vi "Coordinate RND.vi"(8 "Coordinate Min":dbl=10.0, 9 "Coordinate Max":dbl=15.0, 11 "City's":u16=3) -> (1 "City's":cluster{"X":dbl, "Y":dbl}[](graph), 3 "Coordinate[]":T1[](array[typedef]))   [LabVIEW 2015, in "TSP Library.lvlib"]
uses:
  TSP Library.lvlib
  TypeDef/Coordinate.ctl
  <vilib>/Analysis/NI_AALBase.lvlib
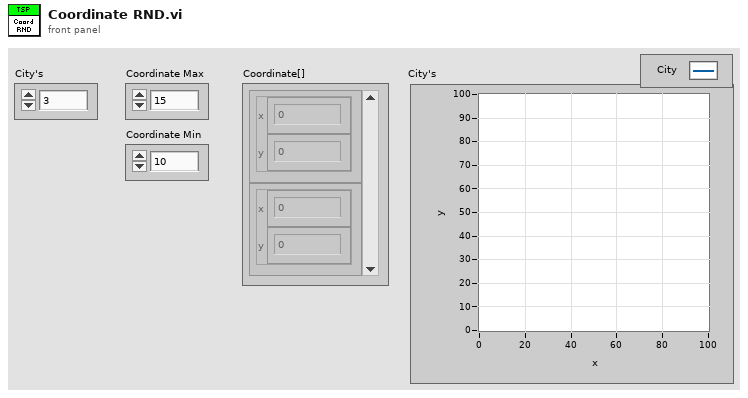
[diagram p1: front panel]
types:
  T1 = typedef "TSP Library.lvlib/Coordinate.ctl" = cluster{"x":dbl, "y":dbl}
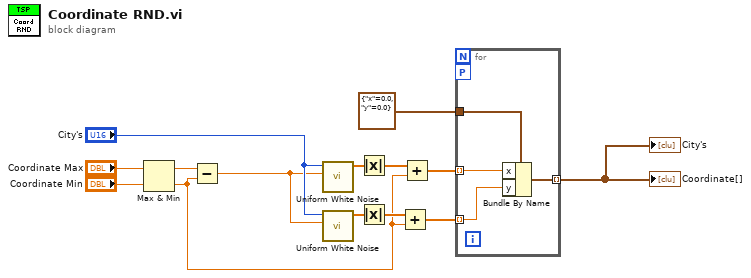
[diagram p0: block diagram]
diagram:
  n1 = Max & Min(x="Coordinate Max", y="Coordinate Min") -> (max(x,y)=w13:dbl, min(x,y)=w2:dbl)
  n2 = Subtract(x=w13, y=w2) -> (x-y=w3:dbl)
  n3 = call <vilib>:"Uniform White Noise.vi"("amplitude"=w3, "samples"="City's") -> ("uniform white noise"=w10:dbl[])  [unwired: 8 in, 1 out]
  n4 = call <vilib>:"Uniform White Noise.vi"("amplitude"=w3, "samples"="City's") -> ("uniform white noise"=w9:dbl[])  [unwired: 8 in, 1 out]
  n5 = Absolute Value(x=w10) -> (abs(x)=w5:dbl[])
  n6 = Absolute Value(x=w9) -> (abs(x)=w4:dbl[])
  n7 = Add(x=w4, y=w2) -> (x+y=w6:dbl[])
  n8 = Add(x=w5, y=w2) -> (x+y=w11:dbl[])
  n9 = for {
    tunnel: w11 -> [w17] mode=indexing
    tunnel: w6 -> [w16] mode=indexing
    tunnel: T1 {"x"=0.0, "y"=0.0} ("Coordinate") -> [w18]
    tunnel: [w15] -> w1 mode=indexing
    workers-P: _ -> [_]
    n10 = Bundle By Name(cluster=w18, "x"=w17, "y"=w16) -> (w15:T1)
  }
  "Coordinate[]" <- w1
  "City's" <- w1
